vi "testYield.vi"() -> ()   [LabVIEW 2018]
panel:
  out "Average Test Time":string
  out "Third Shift":u32
  out "Second Shift":u32
  out "Shortest Test Time":string
  out "First Shift":u32
  out "Tests per Hour":i32
  out "Last Test Time":string
  out "Yield":u32 format="%.1f"
  in  "Boolean":bool
  out "error out":errorcluster
  out "Fails":u32
  out "Passes":u32
  out "Tests":u32
  out "Consecutive Fails":u32
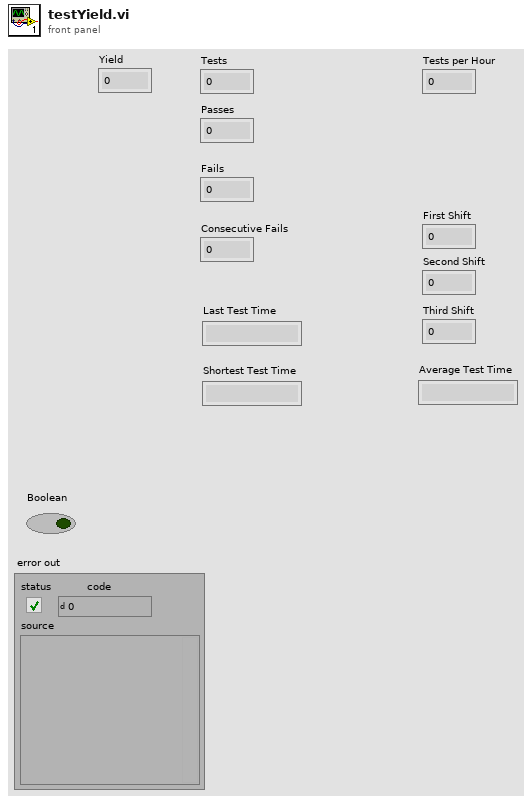
[diagram p1: front panel]
types:
  T1 = cluster{"Tests":i32, "Passes":i32, "Fails":i32, "Consecutive Fails":i32, "Yield":i32, "Last Test Time":string, "Shortest Test Time":string, "Tests per Hour":i32, " First Shift":i32, " Second Shift":i32, "Third Shift ":i32, "Average Test Time":string}
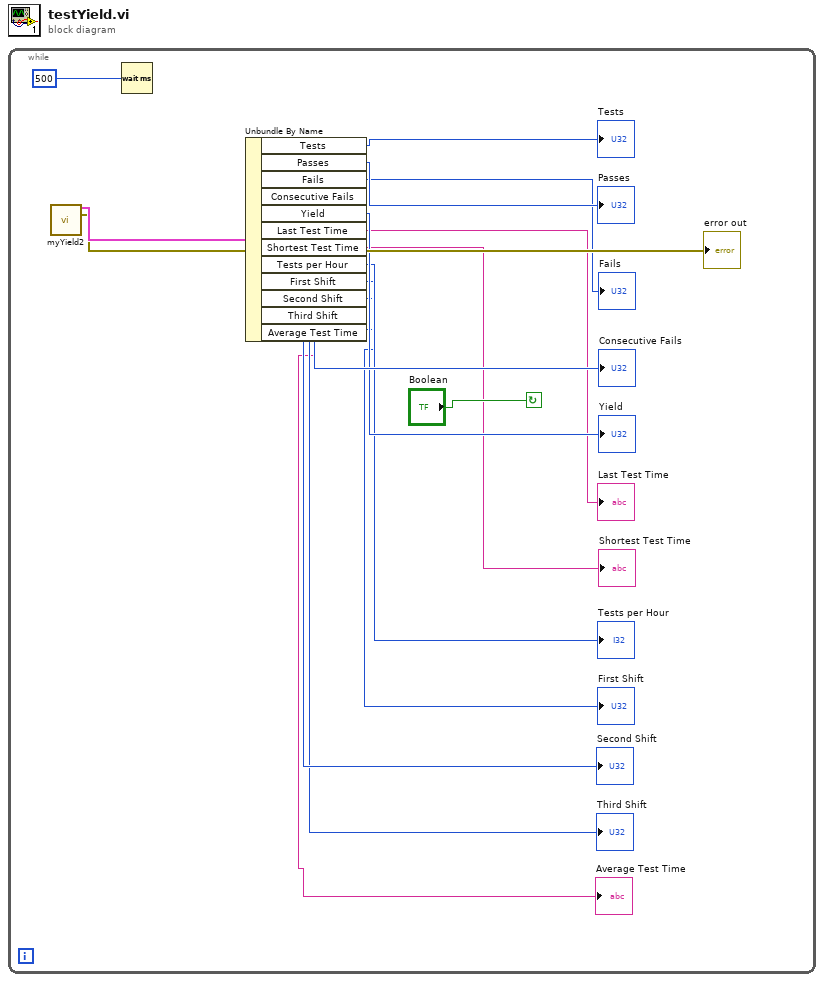
[diagram p0: block diagram]
diagram:
  n1 = while {
    stop <- "Boolean" continue-if-true
    n2 = call "myYield2.vi"() -> ("Results Cluster"=w16:T1, "error out"=→"error out":errorcluster)  [unwired: 14 in]
    n3 = Wait (ms)(milliseconds to wait=500) -> ()  [unwired: 1 out]
    n4 = Unbundle By Name(w16) -> ("Tests"=→"Tests":i32, "Passes"=→"Passes":i32, "Fails"=→"Fails":i32, "Consecutive Fails"=→"Consecutive Fails":i32, "Yield"=→"Yield":i32, "Last Test Time"=→"Last Test Time":string, "Shortest Test Time"=→"Shortest Test Time":string, "Tests per Hour"=→"Tests per Hour":i32, "First Shift"=→"First Shift":i32, "Second Shift"=→"Second Shift":i32, "Third Shift"=→"Third Shift":i32, "Average Test Time"=→"Average Test Time":string)
  }
